vi "WPI_JoystickRatioCurveMapping.vi"(6 "Max Output":dbl=1.0, 7 "Sensitivity":dbl=1.0, 9 "Y axis value (Speed)":dbl, 10 "X axis value (Curve)":dbl) -> (2 "Right Motor Value":dbl, 3 "Left Motor Value":dbl)   [LabVIEW 2017]
doc: "Controls the motor outputs by considering the driving speed independent of the curve rate. This VI is typically used in autonomous mode."
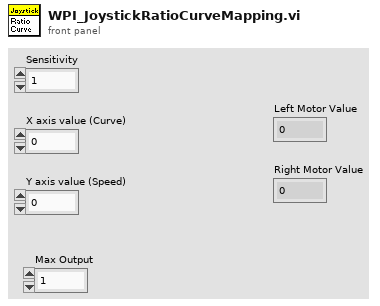
[diagram p1: front panel]
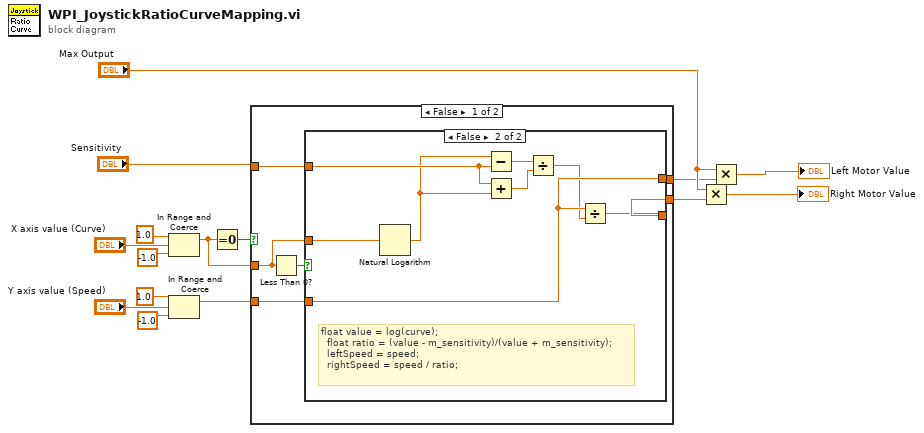
[diagram p0: block diagram]
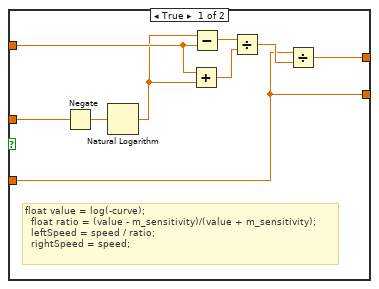
[diagram p2: hidden frame]
diagram:
  n1 = In Range and Coerce(upper limit=1.0, x="X axis value (Curve)", lower limit=-1.0) -> (coerced(x)=w10:dbl)  [unwired: 1 out]
  n2 = In Range and Coerce(upper limit=1.0, x="Y axis value (Speed)", lower limit=-1.0) -> (coerced(x)=w7:dbl)  [unwired: 1 out]
  n3 = Equal To 0?(x=w10) -> (x = 0?=w1:bool)
  n4 = case shown="False" w1 {
    tunnel: w7 -> [w20 w39]
    tunnel: [w17 w39] -> w2
    tunnel: [w16 w39] -> w3
    tunnel: w10 -> [w19 _]
    tunnel: "Sensitivity" -> [w18 _]
    frame False {
      n5 = Less Than 0?(x=w19) -> (x < 0?=w21:bool)
      n6 = case shown="False" w21 {
        tunnel: w18 -> [w27 w38]
        tunnel: w19 -> [w28 w37]
        tunnel: w20 -> [w23 w33]
        tunnel: [w24 w33] -> w17
        tunnel: [w23 w31] -> w16
        frame True {
          # "float value = log(-curve);\n\t\tfloat ratio = (value - m_sensitivity)/(value + m_sensitivity);\n\t\tleftSpeed = speed / ratio;\n\t\trightSpeed = speed;"
          n7 = Negate(x=w28) -> (-x=w26:dbl)
          n8 = Natural Logarithm(1:w26) -> (0:w22:dbl)
          n9 = Add(x=w27, y=w22) -> (x+y=w29:dbl)
          n10 = Subtract(x=w22, y=w27) -> (x-y=w30:dbl)
          n11 = Divide(x=w30, y=w29) -> (x/y=w25:dbl)
          n12 = Divide(x=w23, y=w25) -> (x/y=w24:dbl)
        }
        frame False {
          # "float value = log(curve);\n\t\tfloat ratio = (value - m_sensitivity)/(value + m_sensitivity);\n\t\tleftSpeed = speed;\n\t\trightSpeed = speed / ratio;"
          n13 = Natural Logarithm(1:w37) -> (0:w36:dbl)
          n14 = Subtract(x=w36, y=w38) -> (x-y=w35:dbl)
          n15 = Add(x=w38, y=w36) -> (x+y=w34:dbl)
          n16 = Divide(x=w35, y=w34) -> (x/y=w32:dbl)
          n17 = Divide(x=w33, y=w32) -> (x/y=w31:dbl)
        }
      }
    }
    frame True {
    }
  }
  n18 = Multiply(x="Max Output", y=w3) -> (x*y=→"Right Motor Value":dbl)
  n19 = Multiply(x="Max Output", y=w2) -> (x*y=→"Left Motor Value":dbl)
